vi "Generacion_seno.vi"() -> ()   [LabVIEW 2017]
panel:
  out "Waveform Graph":dbl[](graph)
  in  "file path (use dialog)":path
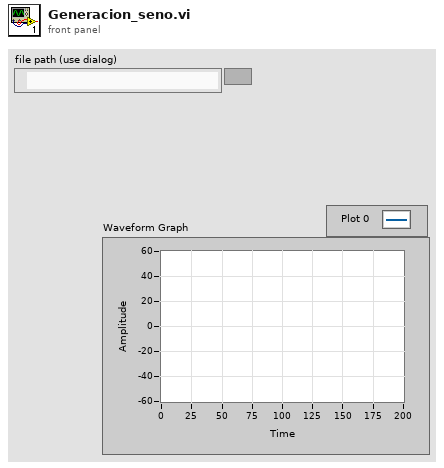
[diagram p1: front panel]
types:
  T1 = enum16{"open", "replace", "create", "open or create", "replace or create", "replace or create with confirmation"}
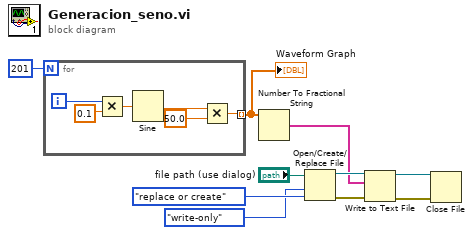
[diagram p0: block diagram]
diagram:
  n1 = for {
    N: 201 -> [_]
    tunnel: [w11] -> w1 mode=indexing
    i -> [w15]
    n2 = Multiply(x=w15, y=0.1) -> (x*y=w14:dbl)
    n3 = Sine(x=w14) -> (sin(x)=w13:dbl)
    n4 = Multiply(x=w13, y=50.0) -> (x*y=w11:dbl)
  }
  "Waveform Graph" <- w1
  n5 = Number To Fractional String(number=w1) -> (F-format string=w5:string[])  [unwired: 3 in]
  n6 = Open/Create/Replace File(file path (use dialog)="file path (use dialog)", operation (0:open)=T1."replace or create", access (0:read/write)=enum16{"read/write", "read-only", "write-only"}."write-only") -> (refnum out=w9:refnum<file>, error out=w8:errorcluster)  [unwired: 3 in, 1 out]
  n7 = Write to Text File(file (use dialog)=w9, text=w5, error in=w8) -> (refnum out=w7:refnum<file>, error out=w6:errorcluster)  [unwired: 1 in, 1 out]
  n8 = Close File(refnum=w7, error in=w6) -> ()  [unwired: 2 out]
